vi "adjust_distance_moved.vi"(1 "Distance Moved":dbl, 2 "Y Change":dbl, 3 "X Change":dbl, 4 "Robot Properties":T1={"Position"=[0.0, 0.0], "Size"=50.0, "Facing"=0.0, "Movement Ratios"=[0.0, -1.0], "Wheel Angle"=0.0}) -> (0 "Adjusted Distance Moved":dbl)   [LabVIEW 2015]
uses:
  Robot.ctl
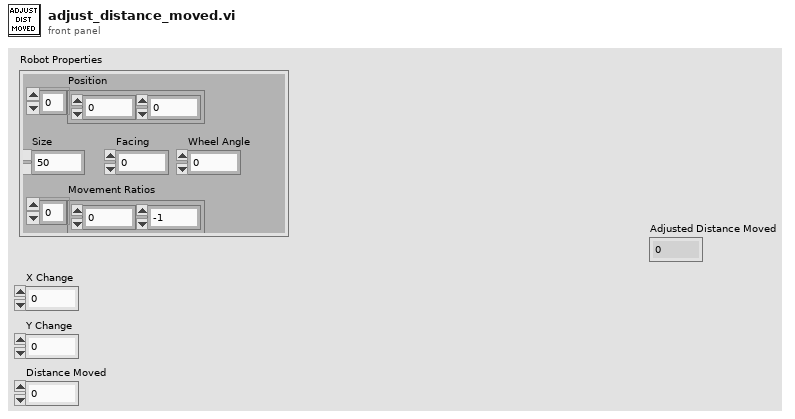
[diagram p1: front panel]
types:
  T1 = typedef "Robot.ctl" = cluster{"Position":dbl[], "Size":dbl, "Facing":dbl, "Movement Ratios":dbl[], "Wheel Angle":dbl}
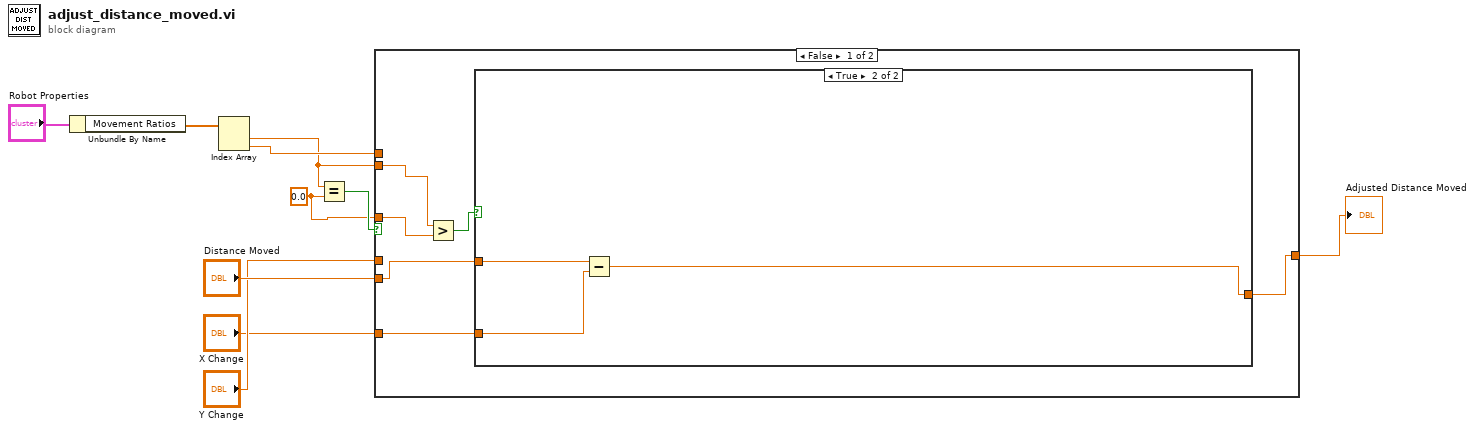
[diagram p0: block diagram]
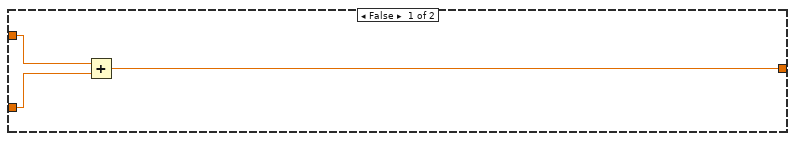
[diagram p2: hidden frame]
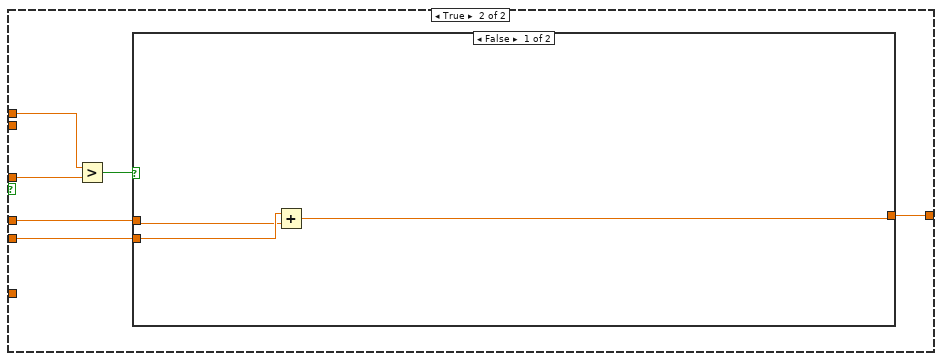
[diagram p3: hidden frame]
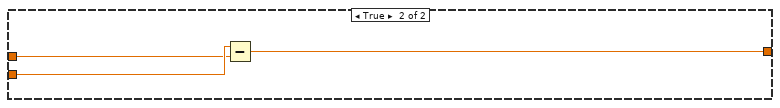
[diagram p4: hidden frame]
diagram:
  w6 = 0.0 ("y")
  n1 = Unbundle By Name("Robot Properties") -> ("Movement Ratios"=w9:dbl[])
  n2 = Index Array(array=w9) -> (element #1=w2:dbl, element #2=w7:dbl)  [unwired: 2 in]
  n3 = Equal?(x=w2, y=w6) -> (x = y?=w8:bool)
  n4 = case shown="False" w8 {
    tunnel: w7 -> [_ w28]
    tunnel: w6 -> [w15 w27]
    tunnel: "Distance Moved" -> [w13 w25]
    tunnel: "Y Change" -> [_ w24]
    tunnel: [w11 w23] -> w3
    tunnel: w2 -> [w16 _]
    tunnel: "X Change" -> [w12 _]
    frame False {
      n5 = Greater?(x=w16, y=w15) -> (0:w14:bool)
      n6 = case shown="True" w14 {
        tunnel: w13 -> [w19 w22]
        tunnel: w12 -> [w18 w21]
        tunnel: [w17 w20] -> w11
        frame False {
          n7 = Add(x=w19, y=w18) -> (x+y=w17:dbl)
        }
        frame True {
          n8 = Subtract(x=w22, y=w21) -> (x-y=w20:dbl)
        }
      }
    }
    frame True {
      n9 = Greater?(x=w28, y=w27) -> (0:w26:bool)
      n10 = case shown="False" w26 {
        tunnel: w25 -> [w31 w34]
        tunnel: w24 -> [w30 w33]
        tunnel: [w29 w32] -> w23
        frame False {
          n11 = Add(x=w31, y=w30) -> (x+y=w29:dbl)
        }
        frame True {
          n12 = Subtract(x=w34, y=w33) -> (x-y=w32:dbl)
        }
      }
    }
  }
  "Adjusted Distance Moved" <- w3
